vi "CRYInsert Data to Listbox.vi"(0 "OrgNames":string[](array[string]), 4 "Type":enum16{"Curves", "Values", "Results", "WFM"}(ring)=enum."Results", 6 "nData":i32[](array[numeric]), 7 "sOption":string, 8 "Waveforms":T2[](array[typedef]) {"Y dB ref" format="%.1f"; "Y axis" items=["Log", "Lin"]; "Y data" items=["dB", "Lin"]; "X data" items=["dB", "Lin"]}, 9 "Results":T3[](array[typedef]) {"Margin" format="%.2f"}, 10 "Values":T1[](array[typedef]) {"Z data" items=["dB", "Lin"]; "X data" items=["dB", "Lin"]; "Y data" items=["dB", "Lin"]; "Z dB ref" format="%.1f"; "Z axis" items=["Log", "Lin"]; "X dB ref" format="%.1f"; "X axis" items=["Log", "Lin"]; "Y axis" items=["Log", "Lin"]; "Y dB ref" format="%.1f"; "Curve"."z" format="%.2f"; "Curve"."y" format="%.2f"; "Curve"."x" format="%.2f"}, 11 "Curves":T1[](array[typedef]) {"Z data" items=["dB", "Lin"]; "X data" items=["dB", "Lin"]; "Y data" items=["dB", "Lin"]; "Z dB ref" format="%.1f"; "Z axis" items=["Log", "Lin"]; "X dB ref" format="%.1f"; "X axis" items=["Log", "Lin"]; "Y axis" items=["Log", "Lin"]; "Y dB ref" format="%.1f"; "Curve"."z" format="%.2f"; "Curve"."y" format="%.2f"; "Curve"."x" format="%.2f"}) -> (3 "Inserted Name Out":string[](array[string]))   [LabVIEW 2013]
uses:
  CRYSystem/Typedef Control/CRYData Cluster.ctl
  CRYSystem/Typedef Control/CRYResult Cluster.ctl
  CRYSystem/Typedef Control/CRYWaveform Cluster.ctl
  Global/CRYCurve Library Global.vi
  CRYProject/CRYProject Editor Global.vi
  CRYMainGlobal.vi
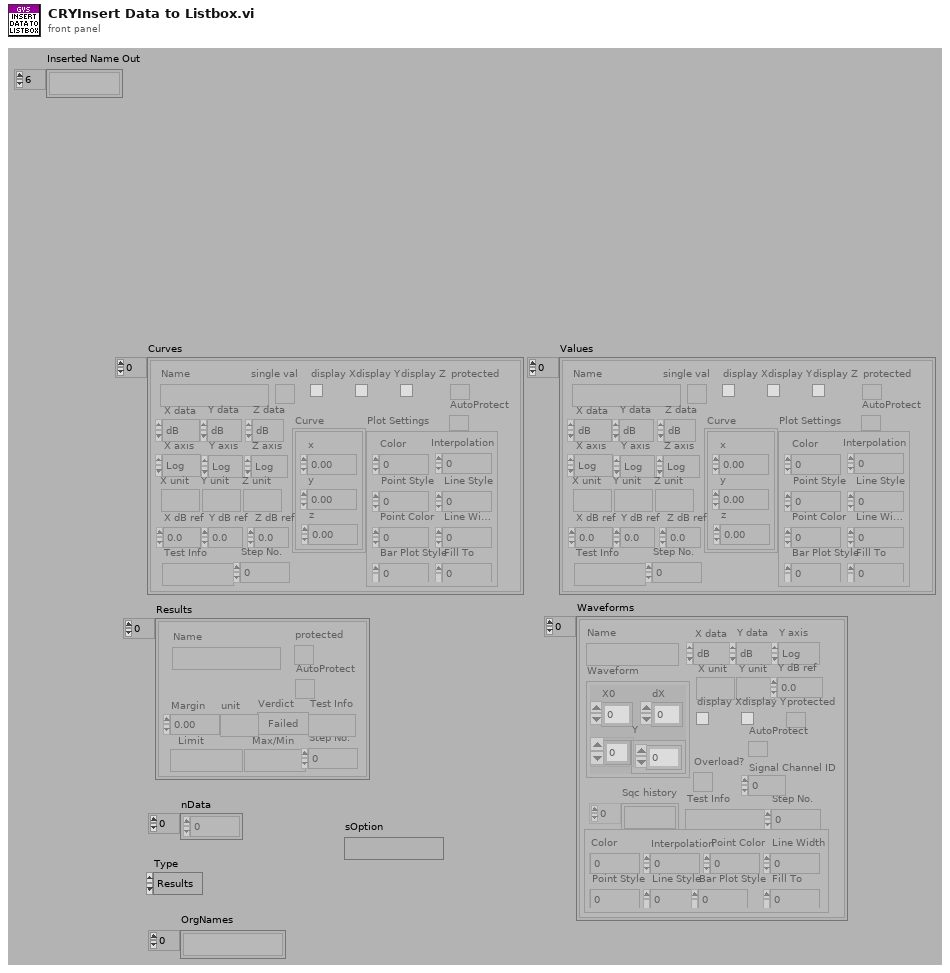
[diagram p1: front panel]
types:
  T1 = typedef "CRYData Cluster.ctl" = cluster{"Name":string, "Curve":cluster{"x":dbl, "y":dbl, "z":dbl}[], "X data":u16, "Y data":u16, "Z data":u16, "X axis":u16, "Y axis":u16, "Z axis":u16, "X unit":string, "Y unit":string, "Z unit":string, "X dB ref":dbl, "Y dB ref":dbl, "Z dB ref":dbl, "single val":bool, "protected":bool, "display X":bool, "display Y":bool, "display Z":bool, "Test Info":string, "Step No.":i32, "Plot Settings":cluster{"Color":u32, "Interpolation":u8, "Point Style":u8, "Line Style":u8, "Point Color":u32, "Line Width":u8, "Bar Plot Style":u8, "Fill To":i16}, "AutoProtect":bool}
  T2 = typedef "CRYWaveform Cluster.ctl" = cluster{"Waveform":cluster{"X0":dbl, "dX":dbl, "Y":sgl[]}, "X data":u16, "Y data":u16, "Y axis":u16, "X unit":string, "Y unit":string, "Y dB ref":dbl, "display Y":bool, "display X":bool, "Overload?":bool, "Test Info":string, "Step No.":i32, "Name":string, "protected":bool, "Sqc history":string[], "Signal Channel ID":i32, "Plot Settings":cluster{"Color":u32, "Interpolation":u8, "Point Style":u8, "Line Style":u8, "Point Color":u32, "Line Width":u8, "Bar Plot Style":u8, "Fill To":i16}, "AutoProtect":bool}
  T3 = typedef "CRYResult Cluster.ctl" = cluster{"Name":string, "Margin":dbl, "unit":string, "Verdict":bool, "Limit":string, "Max/Min":string, "protected":bool, "Step No.":i32, "Test Info":string, "AutoProtect":bool}
  T4 = typedef "CRYCurveLib Info Cluster.ctl" = cluster{"GroupingState":string}
  T5 = typedef "CRYStep.ctl" = cluster{"No.VI":i32, "Category":string, "StepName":string, "Seq setup flattened":string, "Comment":string, "Steps config.":bool[], "Jump config":i32[], "Start":dbl, "Increment":dbl, "Name":string, "Unit":string, "Y data":u16, "Y prefix":string, "Y dB ref":dbl, "Y unit":string, "Repeat State Array":cluster{"Start":dbl, "Increment":dbl, "Count":i32, "Num":i32}[]}
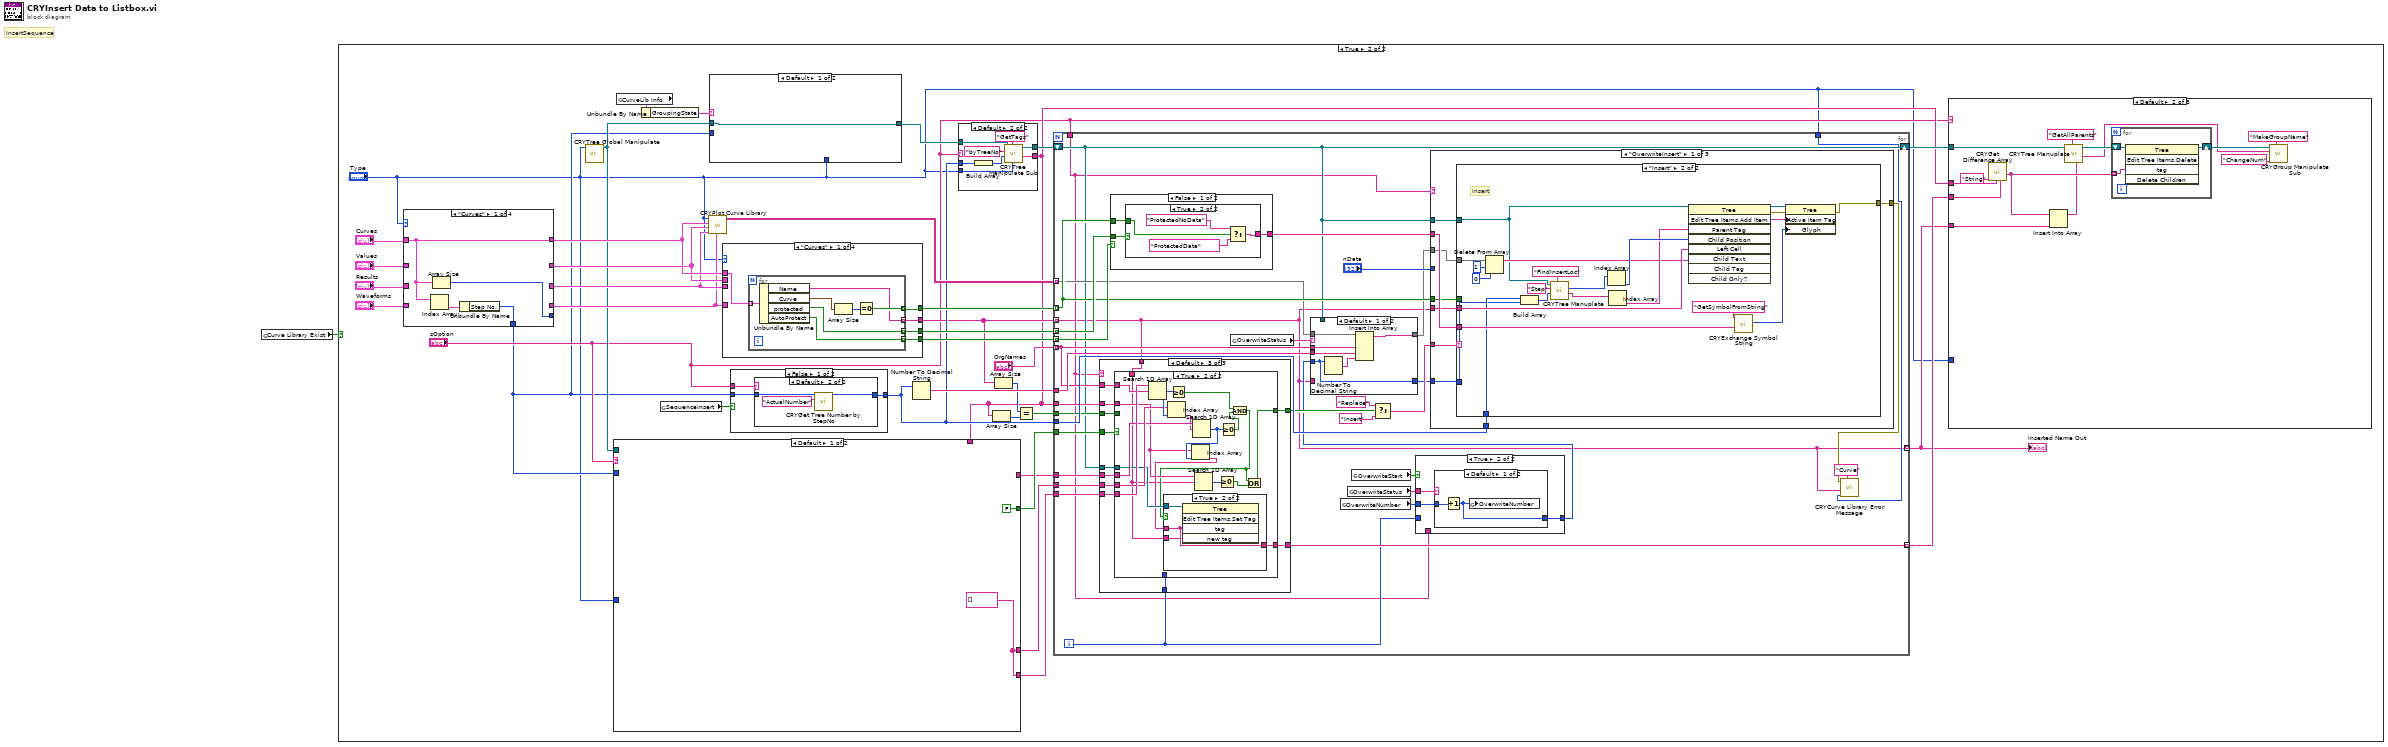
[diagram p0: block diagram]
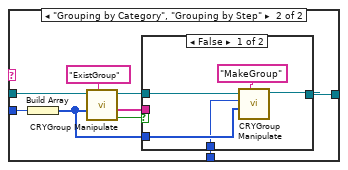
[diagram p3: hidden frame]
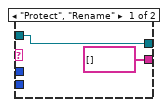
[diagram p5: hidden frame]
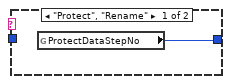
[diagram p6: hidden frame]
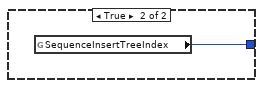
[diagram p7: hidden frame]
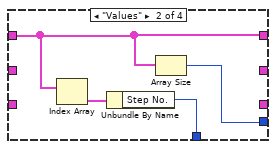
[diagram p8: hidden frame]
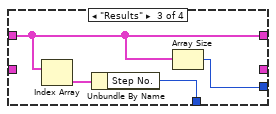
[diagram p9: hidden frame]
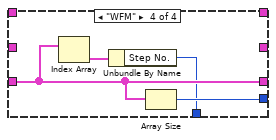
[diagram p10: hidden frame]
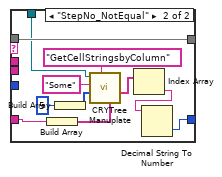
[diagram p11: hidden frame]
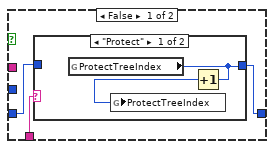
[diagram p12: hidden frame]
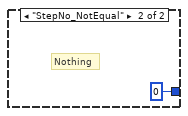
[diagram p14: hidden frame]
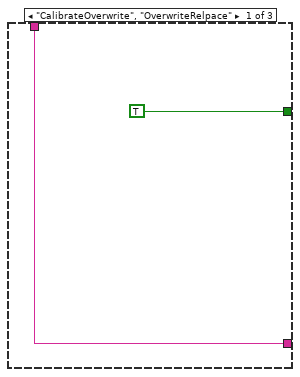
[diagram p15: hidden frame]
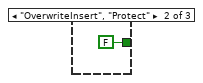
[diagram p16: hidden frame]
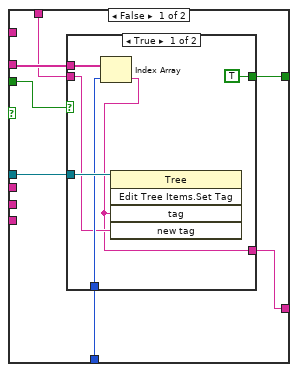
[diagram p17: hidden frame]
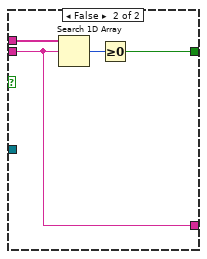
[diagram p18: hidden frame]
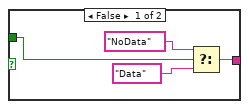
[diagram p20: hidden frame]
diagram:
  # "InsertSequence"
  n1 = global read "CRYCurve Library Global.vi" "Curve Library Exist"() -> (w1:bool)
  n2 = case shown="True" w1 {
    frame False {
    }
    frame True {
      n3 = case shown="\"Curves\"" "Type" {
        tunnel: "Curves" -> [w74 _ _ _]
        tunnel: "Results" -> [_ _ w81 _]
        tunnel: [w74 _ _ _] -> w33
        tunnel: [w75 w79 w83 w87] -> _
        tunnel: [_ _ w81 _] -> w31
        tunnel: "Waveforms" -> [_ _ _ w85]
        tunnel: [_ _ _ w85] -> w30
        tunnel: "Values" -> [_ w77 _ _]
        tunnel: [_ w77 _ _] -> w32
        tunnel: [w72 w76 w80 w84] -> w7
        frame "Curves" {
          n4 = Index Array(array=w74) -> (element=w73:T1)  [unwired: 1 in]
          n5 = Array Size(array=w74) -> (size(s)=w75:i32)
          n6 = Unbundle By Name(w73) -> ("Step No."=w72:i32)
        }
        frame "Values" {
          n7 = Index Array(array=w77) -> (element=w78:T1)  [unwired: 1 in]
          n8 = Unbundle By Name(w78) -> ("Step No."=w76:i32)
          n9 = Array Size(array=w77) -> (size(s)=w79:i32)
        }
        frame "Results" {
          n10 = Index Array(array=w81) -> (element=w82:T3)  [unwired: 1 in]
          n11 = Unbundle By Name(w82) -> ("Step No."=w80:i32)
          n12 = Array Size(array=w81) -> (size(s)=w83:i32)
        }
        frame "WFM" {
          n13 = Index Array(array=w85) -> (element=w86:T2)  [unwired: 1 in]
          n14 = Unbundle By Name(w86) -> ("Step No."=w84:i32)
          n15 = Array Size(array=w85) -> (size(s)=w87:i32)
        }
      }
      n16 = call "CRYTree Global Manipulate.vi"("Type In"="Type") -> ("Tree/Curve Tree"=w13:refnum<vi>)  [unwired: 7 in, 3 out]
      n17 = global read "CRYCurve Library Global.vi" "CurveLib Info"() -> (w9:T4)
      n18 = Unbundle By Name(w9) -> ("GroupingState"=w8:string)
      n19 = global read "CRYProject Editor Global.vi" "SequenceInsert"() -> (w14:bool)
      n20 = call "CRYPlot Curve Library.vi"("Waveform"=w30, "Results"=w31, "Values"=w32, "Curves"=w33, "Type"="Type") -> ("PlotStrings"=w34:string[][])  [unwired: 6 in]
      n21 = case shown="Default" w8 {
        tunnel: w13 -> [w38 w44]
        tunnel: [w38 w42] -> w12
        tunnel: w7 -> [_ w41]
        tunnel: "Type" -> [_ w39]
        frame Default {
        }
        frame "Grouping by Category", "Grouping by Step" {
          n22 = Build Array(w41) -> (w40:i32[])
          n23 = call "CRYGroup Manipulate.vi"("sAction"="ExistGroup", "nData"=w40, "Tree in"=w44) -> ("bData out"=w47:bool, "sData Out"=w43:string[], "Tree Out"=w46:refnum<vi>)  [unwired: 5 in, 1 out]
          n24 = case shown="False" w47 {
            tunnel: w46 -> [w51 w53]
            tunnel: w43 -> [_ _]
            tunnel: [w50 w53] -> w42
            tunnel: w40 -> [w49 _]
            tunnel: w39 -> [w48 _]
            frame False {
              n25 = call "CRYGroup Manipulate.vi"("sAction"="MakeGroup", "nData"=w49, "Type"=w48, "Tree in"=w51) -> ("Tree Out"=w50:refnum<vi>)  [unwired: 4 in, 3 out]
            }
            frame True {
            }
          }
        }
      }
      n26 = case shown="\"Curves\"" "Type" {
        tunnel: [w400 w412 w425 w439] -> w37
        tunnel: [w399 w411 w424 w438] -> w19
        tunnel: [w398 w410 w423 w437] -> w36
        tunnel: [w397 w409 w422 w436] -> w35
        tunnel: w33 -> [w396 _ _ _]
        tunnel: w32 -> [_ w408 _ _]
        tunnel: w31 -> [_ _ w421 _]
        tunnel: w30 -> [_ _ _ w435]
        frame "Curves" {
          n27 = for {
            tunnel: w396 -> [w406] mode=indexing
            tunnel: [w405] -> w400 mode=indexing
            tunnel: [w401] -> w399 mode=indexing
            tunnel: [w403] -> w398 mode=indexing
            tunnel: [w402] -> w397 mode=indexing
            n28 = Unbundle By Name(w406) -> ("Name"=w401:string, "Curve"=w407:cluster{"x":dbl, "y":dbl, "z":dbl}[], "protected"=w403:bool, "AutoProtect"=w402:bool)
            n29 = Array Size(array=w407) -> (size(s)=w404:i32)
            n30 = Equal To 0?(x=w404) -> (x = 0?=w405:bool)
          }
        }
        frame "Values" {
          n31 = for {
            tunnel: w408 -> [w419] mode=indexing
            tunnel: [w416] -> w412 mode=indexing
            tunnel: [w413] -> w411 mode=indexing
            tunnel: [w415] -> w410 mode=indexing
            tunnel: [w414] -> w409 mode=indexing
            n32 = Unbundle By Name(w419) -> ("Name"=w413:string, "Curve"=w420:cluster{"x":dbl, "y":dbl, "z":dbl}[], "protected"=w415:bool, "AutoProtect"=w414:bool)
            n33 = Array Size(array=w420) -> (size(s)=w417:i32)
            n34 = Equal?(x=w417, y=0) -> (x = y?=w416:bool)
          }
        }
        frame "Results" {
          n35 = for {
            tunnel: w421 -> [w434] mode=indexing
            tunnel: [w433] -> w425 mode=indexing
            tunnel: [w426] -> w424 mode=indexing
            tunnel: [w428] -> w423 mode=indexing
            tunnel: [w427] -> w422 mode=indexing
            n36 = Unbundle By Name(w434) -> ("Name"=w426:string, "Margin"=w432:dbl, "protected"=w428:bool, "AutoProtect"=w427:bool)
            n37 = Format Value(format string="%f", value (0)=w432) -> (output string=w429:string)  [unwired: 1 in]
            n38 = Equal?(x="NaN", y=w429) -> (x = y?=w433:bool)
          }
        }
        frame "WFM" {
          n39 = for {
            tunnel: w435 -> [w444] mode=indexing
            tunnel: [w443] -> w439 mode=indexing
            tunnel: [w440] -> w438 mode=indexing
            tunnel: [w442] -> w437 mode=indexing
            tunnel: [w441] -> w436 mode=indexing
            n40 = Unbundle By Name(w444) -> ("Name"=w440:string, "Waveform.Y"=w446:sgl[], "protected"=w442:bool, "AutoProtect"=w441:bool)
            n41 = Array Size(array=w446) -> (size(s)=w447:i32)
            n42 = Equal?(x=w447, y=0) -> (x = y?=w443:bool)
          }
        }
      }
      n43 = case shown="False" w14 {
        tunnel: "sOption" -> [w66 _]
        tunnel: [w65 w71] -> w26
        tunnel: w7 -> [w64 _]
        frame False {
          n44 = case shown="Default" w66 {
            tunnel: w64 -> [_ w70]
            tunnel: [w67 w69] -> w65
            frame "Protect", "Rename" {
              n45 = global read "CRYCurve Library Global.vi" "ProtectDataStepNo"() -> (w67:i32)
            }
            frame Default {
              n46 = call "CRYGet Tree Number by StepNo.vi"("sOption"="ActualNumber", "Step Setup VI No"=w70) -> ("Number in Tree"=w69:i32)  [unwired: 8 in, 1 out]
            }
          }
        }
        frame True {
          n47 = global read "CRYProject Editor Global.vi" "SequenceInsertTreeIndex"() -> (w71:i32)
        }
      }
      n48 = Number To Decimal String(number=w26) -> (decimal integer string=w27:string)  [unwired: 1 in]
      n49 = case shown="Default" "sOption" {
        tunnel: "Type" -> [_ w63]
        tunnel: [w55 w59] -> w29
        tunnel: w26 -> [_ w58]
        tunnel: [string[] [] ("sData Out") w57] -> w15
        tunnel: w12 -> [w55 w56]
        frame "Protect", "Rename" {
        }
        frame Default {
          n50 = Build Array(w58) -> (w60:i32[])
          n51 = call "CRYTree Manipulate Sub.vi"("Type"=w63, "sAction"="GetTags", "nData"=w60, "sOption"="byTreeNo", "Tree in"=w56) -> ("sData Out"=w57:string[], "Tree Out"=w59:refnum<vi>)  [unwired: 2 in, 3 out]
        }
      }
      n52 = case shown="Default" "sOption" {
        tunnel: w7 -> [_ w461]
        tunnel: [w448 w460] -> w23
        tunnel: [FALSE w459] -> w25
        tunnel: [w448 w458] -> w22
        tunnel: w13 -> [_ w455]
        tunnel: [_ w452] -> w21
        tunnel: "Type" -> [_ w451]
        tunnel: w15 -> [_ w450]
        frame Default {
          w448 = string[] [] ("Changed Curve State")
        }
        frame "Apply", "StepOK" {
          n53 = call "CRYGet Current TS Steps.vi"() -> ("Steps"=w462:T5[])  [unwired: 7 in, 4 out]
          n54 = for {
            tunnel: w462 -> [w509] mode=indexing
            tunnel: w461 -> [w507]
            tunnel: [w502] -> w459
            stop <- w502 stop-if-true
            n55 = Unbundle By Name(w509) -> ("No.VI"=w508:i32, "Category"=w505:string)
            n56 = Equal?(x=w507, y=w508) -> (x = y?=w506:bool)
            n57 = Equal?(x=w505, y="Analysis") -> (x = y?=w500:bool)
            n58 = Equal?(x=w505, y="Acqusition") -> (x = y?=w501:bool)
            n59 = Or(x=w500, y=w501) -> (x .or. y?=w499:bool)
            n60 = And(x=w506, y=w499) -> (x .and. y?=w502:bool)
          }
          n61 = case shown="True" w459 {
            tunnel: [_ w463] -> w460
            tunnel: [_ w464] -> w458
            tunnel: w451 -> [_ w467]
            frame False {
            }
            frame True {
              w465 = string[] [] ("Changed Curve State")
              n62 = global read "CRYMainGlobal.vi" "Changed Curve State"() -> (w466:string[][])
              n63 = for {
                tunnel: w467 -> [w486]
                tunnel: w466 -> [w481] mode=indexing
                shift-right: [w470] -> w464
                shift-left: w465 -> [w471]
                shift-right: [w468] -> w463
                shift-left: w465 -> [w469]
                # "New Names"
                # "Old Names"
                n64 = case shown="\"WFM\"" w486 {
                  tunnel: ["Curve" ("Custom Curve Names") "Value" ("Custom Curve Names") "Result" ("Custom Curve Names") "Wave" ("Custom Curve Names")] -> w480
                  frame "Curves", Default {
                  }
                  frame "Values" {
                  }
                  frame "Results" {
                  }
                  frame "WFM" {
                  }
                }
                n65 = Index Array(array=w481, index #1=3 ("index"), index #2=2 ("index"), index #3=0 ("index"), index #4=1 ("index")) -> (element #1=w479:string, element #2=w478:string, element #3=w473:string, element #4=w472:string)
                n66 = Equal?(x=w480, y=w479) -> (x = y?=w476:bool)
                n67 = Equal?(x="R", y=w478) -> (x = y?=w475:bool)
                n68 = And(x=w476, y=w475) -> (x .and. y?=w474:bool)
                n69 = case shown="True" w474 {
                  tunnel: w473 -> [_ w490]
                  tunnel: w472 -> [_ w489]
                  tunnel: w471 -> [w488 w494]
                  tunnel: [w488 w493] -> w470
                  tunnel: w469 -> [w487 w492]
                  tunnel: [w487 w491] -> w468
                  frame False {
                  }
                  frame True {
                    n70 = Insert Into Array(array=w492, new element=w489) -> (w491:string[])  [unwired: 1 in]
                    n71 = Insert Into Array(array=w494, new element=w490) -> (w493:string[])  [unwired: 1 in]
                  }
                }
              }
            }
          }
          n72 = Build Array(3) -> (w453:i32[])
          n73 = call "CRYTree Manuplate.vi"("sData"=w450, "sAction"="GetCellStringsbyColumn", "nData"=w453, "sOption"="Some", "Tree in"=w455) -> ("sData Out"=w452:string[])  [unwired: 3 in, 3 out]
        }
      }
      n74 = Array Size(array=w15) -> (size(s)=w17:i32)
      n75 = Array Size(array=w19) -> (size(s)=w18:i32)
      n76 = Equal?(x=w18, y=w17) -> (x = y?=w16:bool)
      n77 = for {
        tunnel: [w89] -> w10 mode=indexing
        tunnel: w34 -> [w95] mode=indexing
        tunnel: w37 -> [w119] mode=indexing
        tunnel: w19 -> [w89] mode=indexing
        tunnel: w36 -> [w120] mode=indexing
        tunnel: w35 -> [w121] mode=indexing
        shift-right: [w93] -> w28
        shift-left: w29 -> [w93]
        tunnel: "OrgNames" -> [w109] mode=indexing
        tunnel: w27 -> [w117]
        tunnel: w26 -> [w113]
        tunnel: w15 -> [w105]
        tunnel: "sOption" -> [w92]
        tunnel: w25 -> [w110]
        tunnel: w23 -> [w107]
        tunnel: w22 -> [w108]
        tunnel: w21 -> [w106]
        tunnel: [w104] -> w20 mode=indexing
        tunnel: w16 -> [w103]
        tunnel: "Type" -> [w90]
        i -> [w99]
        n78 = case shown="Default" w92 {
          tunnel: w105 -> [_ _ w159]
          tunnel: w89 -> [w151 _ w158]
          tunnel: [TRUE FALSE w157] -> w112
          tunnel: w110 -> [_ _ w165]
          tunnel: w109 -> [_ _ w164]
          tunnel: w108 -> [_ _ w163]
          tunnel: w107 -> [_ _ w162]
          tunnel: w106 -> [_ _ w161]
          tunnel: w93 -> [_ _ w160]
          tunnel: [w151 _ w156] -> w104
          tunnel: w103 -> [_ _ w155]
          tunnel: w99 -> [_ _ w154]
          frame "CalibrateOverwrite", "OverwriteRelpace" {
          }
          frame "OverwriteInsert", "Protect" {
          }
          frame Default {
            n79 = case shown="True" w165 {
              tunnel: w159 -> [w172 w188]
              tunnel: w158 -> [w170 w184]
              tunnel: w164 -> [_ w199]
              tunnel: w163 -> [_ w197]
              tunnel: w162 -> [_ w200]
              tunnel: w161 -> [_ w195]
              tunnel: w160 -> [w169 w191]
              tunnel: [w171 w185] -> w157
              tunnel: [w166 w183] -> w156
              tunnel: w155 -> [w168 _]
              tunnel: w154 -> [w167 _]
              frame False {
                n80 = case shown="True" w168 {
                  tunnel: w172 -> [w176 w181]
                  tunnel: [TRUE w180] -> w171
                  tunnel: w170 -> [w174 w179]
                  tunnel: w169 -> [w178 _]
                  tunnel: w167 -> [w175 _]
                  tunnel: [w173 w179] -> w166
                  frame True {
                    n81 = Index Array(array=w176, index=w175) -> (element=w173:string)
                    n82 = invoke class="Tree" method="Edit Tree Items.Set Tag"(reference=w178, "tag"=w173, "new tag"=w174) -> ()  [unwired: 2 in, 5 out]
                  }
                  frame False {
                    n83 = Search 1D Array(1D array=w181, element=w179) -> (index of element=w182:i32)  [unwired: 1 in]
                    n84 = Greater Or Equal To 0?(x=w182) -> (x >= 0?=w180:bool)
                  }
                }
              }
              frame True {
                n85 = Search 1D Array(1D array=w200, element=w199) -> (index of element=w198:i32)  [unwired: 1 in]
                n86 = Index Array(array=w197, index=w198) -> (element=w194:string)
                n87 = Greater Or Equal To 0?(x=w198) -> (x >= 0?=w196:bool)
                n88 = Search 1D Array(1D array=w195, element=w194) -> (index of element=w192:i32)  [unwired: 1 in]
                n89 = Index Array(array=w188, index=w192) -> (element=w190:string)
                n90 = Search 1D Array(1D array=w188, element=w184) -> (index of element=w189:i32)  [unwired: 1 in]
                n91 = Greater Or Equal To 0?(x=w189) -> (x >= 0?=w187:bool)
                n92 = Greater Or Equal To 0?(x=w192) -> (x >= 0?=w193:bool)
                n93 = And(x=w196, y=w193) -> (x .and. y?=w186:bool)
                n94 = case shown="True" w186 {
                  tunnel: w191 -> [_ w204]
                  tunnel: w190 -> [_ w203]
                  tunnel: w184 -> [w201 w202]
                  tunnel: [w201 w203] -> w183
                  frame False {
                  }
                  frame True {
                    n95 = invoke class="Tree" method="Edit Tree Items.Set Tag"(reference=w204, "tag"=w203, "new tag"=w202) -> ()  [unwired: 2 in, 5 out]
                  }
                }
                n96 = Or(x=w186, y=w187) -> (x .or. y?=w185:bool)
              }
            }
          }
        }
        n97 = case shown="False" w121 {
          tunnel: w119 -> [w206 w219]
          tunnel: [w205 w218] -> w118
          tunnel: w120 -> [w207 _]
          frame False {
            n98 = case shown="True" w207 {
              tunnel: w206 -> [w211 w215]
              tunnel: [w210 w214] -> w205
              frame False {
                n99 = Select(t="NoData" ("name or relative path"), s=w211, f="Data" ("name or relative path")) -> (s? t:f=w210:string)
              }
              frame True {
                n100 = Select(t="ProtectedNoData" ("name or relative path"), s=w215, f="ProtectedData" ("name or relative path")) -> (s? t:f=w214:string)
              }
            }
          }
          frame True {
            # "AutoProtect"
            n101 = Select(t="AutoProtectNoData" ("name or relative path"), s=w219, f="AutoProtectData" ("name or relative path")) -> (s? t:f=w218:string)
          }
        }
        n102 = global read "CRYCurve Library Global.vi" "OverwriteStatus"() -> (w97:string)
        n103 = global read "CRYCurve Library Global.vi" "OverwriteNumber"() -> (w100:i32)
        n104 = global read "CRYCurve Library Global.vi" "OverwriteStatus"() -> (w101:string)
        n105 = global read "CRYCurve Library Global.vi" "OverwriteStart"() -> (w102:bool)
        n106 = Select(t="Replace", s=w112, f="Insert" ("sOption")) -> (s? t:f=w114:string)
        n107 = case shown="True" w102 {
          tunnel: w101 -> [_ w147]
          tunnel: w100 -> [_ w146]
          tunnel: w99 -> [w140 _]
          tunnel: [w141 w145] -> w98
          tunnel: w92 -> [w139 _]
          frame False {
            n108 = case shown="\"Protect\"" w139 {
              tunnel: [w143 w144] -> w141
              tunnel: w140 -> [_ w144]
              frame "Protect" {
                n109 = global read "CRYCurve Library Global.vi" "ProtectTreeIndex"() -> (w143:i32)
                n110 = Increment(x=w143) -> (x+1=w142:i32)
                n111 = global write "CRYCurve Library Global.vi" "ProtectTreeIndex"(w142) -> ()
              }
              frame Default {
              }
            }
          }
          frame True {
            n112 = case shown="Default" w147 {
              tunnel: w146 -> [w149 _]
              tunnel: [w148 0] -> w145
              frame Default {
                n113 = Increment(x=w149) -> (x+1=w148:i32)
                n114 = global write "CRYCurve Library Global.vi" "OverwriteNumber"(w148) -> ()
              }
              frame "StepNo_NotEqual" {
                # "Nothing"
              }
            }
          }
        }
        n115 = case shown="Default" w97 {
          tunnel: w117 -> [w127 _]
          tunnel: w109 -> [w125 _]
          tunnel: w98 -> [w122 _]
          tunnel: [w124 w138] -> w96
          tunnel: w95 -> [w123 w138]
          tunnel: [w122 w128] -> w94
          tunnel: w89 -> [_ w133]
          tunnel: w93 -> [_ w131]
          frame Default {
            n116 = Number To Decimal String(number=w122) -> (decimal integer string=w126:string)  [unwired: 1 in]
            n117 = Insert Into Array(array=w123, new element #1=w125, new element #2=w127, new element #3=w126) -> (w124:string[])  [unwired: 1 in]
          }
          frame "StepNo_NotEqual" {
            n118 = Build Array(w133) -> (w132:string[])
            n119 = Build Array(5) -> (w134:i32[])
            n120 = call "CRYTree Manuplate.vi"("sData"=w132, "sAction"="GetCellStringsbyColumn", "nData"=w134, "sOption"="Some", "Tree in"=w131) -> ("sData Out"=w130:string[])  [unwired: 3 in, 3 out]
            n121 = Index Array(array=w130) -> (element=w129:string)  [unwired: 1 in]
            n122 = Decimal String To Number(string=w129) -> (number=w128:i32)  [unwired: 2 in, 1 out]
          }
        }
        n123 = case shown="\"OverwriteInsert\"" w92 {
          tunnel: w118 -> [w228 w295 _]
          tunnel: w96 -> [w227 w294 w381]
          tunnel: w119 -> [w226 w293 _]
          tunnel: w114 -> [w222 w292 _]
          tunnel: w93 -> [w225 w291 w383]
          tunnel: w89 -> [w224 w290 _]
          tunnel: w113 -> [w223 w289 _]
          tunnel: "nData" -> [_ _ w386]
          tunnel: w94 -> [w221 w288 w380]
          tunnel: [w220 w287 w377] -> w91
          frame "OverwriteInsert" {
            n124 = case shown="\"Insert\"" w222 {
              tunnel: w227 -> [w237 w269]
              tunnel: w228 -> [w242 w282]
              tunnel: w226 -> [w244 _]
              tunnel: w225 -> [w243 w267]
              tunnel: w224 -> [w232 w284]
              tunnel: w223 -> [_ w280]
              tunnel: w221 -> [_ w279]
              tunnel: [w229 w265] -> w220
              frame "Replace", Default {
                n125 = property on="Property Node" class="Tree"(reference=w243, "Active Item Tag"=w232) -> (reference out=w240:refnum<vi>, error out=w231:errorcluster, "Glyph"=w239:i32)  [unwired: 1 in]
                n126 = call "CRYExchange Symbol String.vi"("nData"=w239, "sAction"="GetStringFromSymbol") -> ("sData out"=w235:string)  [unwired: 8 in, 1 out]
                n127 = case shown="\"DataView\", \"NoDataView\"" w235 {
                  tunnel: w244 -> [_ w249 w253 w257]
                  tunnel: [w245 w248 w252 w256] -> w233
                  tunnel: w242 -> [w245 _ _ _]
                  frame Default {
                  }
                  frame "DataView", "NoDataView" {
                    n128 = Select(t="NoDataView" ("name or relative path"), s=w249, f="DataView" ("name or relative path")) -> (s? t:f=w248:string)
                  }
                  frame "AutoProtectDataView", "AutoProtectNoDataView" {
                    n129 = Select(t="AutoProtectNoDataView" ("name or relative path"), s=w253, f="AutoProtectDataView" ("name or relative path")) -> (s? t:f=w252:string)
                  }
                  frame "ProtectedDataView", "ProtectedNoDataView" {
                    n130 = Select(t="ProtectedNoDataView" ("name or relative path"), s=w257, f="ProtectedDataView" ("name or relative path")) -> (s? t:f=w256:string)
                  }
                }
                n131 = call "CRYExchange Symbol String.vi"("sData"=w233, "sAction"="GetSymbolFromString") -> ("nData out"=w238:i32)  [unwired: 8 in, 1 out]
                n132 = property on="Property Node" class="Tree"(reference=w240, error in=w231, "Active Item Tag"=w232, "Glyph"=w238) -> (reference out=w241:refnum<vi>, error out=w230:errorcluster)
                n133 = for {
                  shift-right: [w263] -> _
                  shift-left: w241 -> [w264]
                  tunnel: w232 -> [w262]
                  tunnel: w237 -> [w260] mode=indexing
                  shift-right: [w258] -> w229
                  shift-left: w230 -> [w259]
                  i -> [w261]
                  n134 = property on="Property Node" class="Tree"(reference=w264, error in=w259, "Active Item Tag"=w262, "ActiveColNum"=w261, "Cell String"=w260) -> (reference out=w263:refnum<vi>, error out=w258:errorcluster)
                }
              }
              frame "Insert" {
                # "Insert"
                n135 = Delete From Array(array=w269, length=1, index=0) -> (array with subset deleted=w268:string[])  [unwired: 1 out]
                n136 = Build Array(w280, w279) -> (w274:i32[])
                n137 = call "CRYTree Manuplate.vi"("sAction"="FindInsertLoc", "nData"=w274, "sOption"="Step", "Tree in"=w267) -> ("sData Out"=w275:string[], "nData Out"=w276:i32[])  [unwired: 4 in, 2 out]
                n138 = Index Array(array=w276) -> (element=w273:i32)  [unwired: 1 in]
                n139 = Index Array(array=w275) -> (element=w272:string)  [unwired: 1 in]
                n140 = invoke class="Tree" method="Edit Tree Items.Add Item"(reference=w267, "Parent Tag"=w272, "Child Position"=w273, "Left Cell"=w284, "Child Text"=w268) -> (reference out=w285:refnum<vi>, error out=w266:errorcluster, "Edit Tree Items:Add Item"=w286:string)  [unwired: 4 in, 6 out]
                n141 = call "CRYExchange Symbol String.vi"("sData"=w282, "sAction"="GetSymbolFromString") -> ("nData out"=w281:i32)  [unwired: 8 in, 1 out]
                n142 = property class="Tree"(reference=w285, error in=w266, "Active Item Tag"=w286, "Glyph"=w281) -> (error out=w265:errorcluster)  [unwired: 1 out]
              }
            }
          }
          frame Default {
            n143 = case shown="\"Replace\"" w292 {
              tunnel: w294 -> [w318 w363]
              tunnel: w295 -> [w322 w372]
              tunnel: w293 -> [w323 _]
              tunnel: w291 -> [w308 w370]
              tunnel: w290 -> [w297 w374]
              tunnel: w289 -> [w312 w366]
              tunnel: w288 -> [w305 w361]
              tunnel: [w296 w354] -> w287
              frame "Replace" {
                n144 = Build Array(w312, w305) -> (w317:i32[])
                n145 = Build Array(w297) -> (w309:string[])
                n146 = call "CRYTree Manuplate.vi"("sData"=w309, "sAction"="FindInsertLoc", "nData"=w317, "sOption"="MovebyReplace", "Tree in"=w308) -> ("bResult Out"=w311:bool, "sData Out"=w316:string[], "nData Out"=w315:i32[], "Tree Out"=w306:refnum<vi>)  [unwired: 3 in]
                n147 = property on="Property Node" class="Tree"(reference=w306, "Active Item Tag"=w297) -> (reference out=w310:refnum<vi>, error out=w300:errorcluster, "Glyph"=w320:i32)  [unwired: 1 in]
                n148 = call "CRYExchange Symbol String.vi"("nData"=w320, "sAction"="GetStringFromSymbol") -> ("sData out"=w303:string)  [unwired: 8 in, 1 out]
                n149 = case shown="\"ProtectedDataView\", \"ProtectedNoDataView\"" w303 {
                  tunnel: w323 -> [_ w328 w332 w336]
                  tunnel: [w324 w327 w331 w335] -> w301
                  tunnel: w322 -> [w324 _ _ _]
                  frame Default {
                  }
                  frame "DataView", "NoDataView" {
                    n150 = Select(t="NoDataView" ("name or relative path"), s=w328, f="DataView" ("name or relative path")) -> (s? t:f=w327:string)
                  }
                  frame "AutoProtectDataView", "AutoProtectNoDataView" {
                    n151 = Select(t="AutoProtectNoDataView" ("name or relative path"), s=w332, f="AutoProtectDataView" ("name or relative path")) -> (s? t:f=w331:string)
                  }
                  frame "ProtectedDataView", "ProtectedNoDataView" {
                    n152 = Select(t="ProtectedNoDataView" ("name or relative path"), s=w336, f="ProtectedDataView" ("name or relative path")) -> (s? t:f=w335:string)
                  }
                }
                n153 = call "CRYExchange Symbol String.vi"("sData"=w301, "sAction"="GetSymbolFromString") -> ("nData out"=w319:i32)  [unwired: 8 in, 1 out]
                n154 = property on="Property Node" class="Tree"(reference=w310, error in=w300, "Active Item Tag"=w297, "Glyph"=w319) -> (reference out=w321:refnum<vi>, error out=w299:errorcluster)
                n155 = for {
                  shift-right: [w352] -> w307
                  shift-left: w321 -> [w353]
                  tunnel: w297 -> [w351]
                  tunnel: w318 -> [w349] mode=indexing
                  shift-right: [w347] -> w298
                  shift-left: w299 -> [w348]
                  i -> [w350]
                  n156 = property on="Property Node" class="Tree"(reference=w353, error in=w348, "Active Item Tag"=w351, "ActiveColNum"=w350, "Cell String"=w349) -> (reference out=w352:refnum<vi>, error out=w347:errorcluster)
                }
                n157 = case shown="False" w311 {
                  tunnel: w316 -> [w345 _]
                  tunnel: w315 -> [w344 _]
                  tunnel: w297 -> [w341 _]
                  tunnel: w307 -> [w339 _]
                  tunnel: w298 -> [w338 w346]
                  tunnel: [w337 w346] -> w296
                  frame False {
                    n158 = Index Array(array=w345) -> (element=w342:string)  [unwired: 1 in]
                    n159 = Index Array(array=w344) -> (element=w343:i32)  [unwired: 1 in]
                    n160 = invoke class="Tree" method="Edit Tree Items.Move Item"(reference=w339, error in=w338, "tag"=w341, "New Parent"=w342, "New Position"=w343, "Carry Children"=TRUE ("Carry Children?")) -> (error out=w337:errorcluster)  [unwired: 1 in, 6 out]
                  }
                  frame True {
                  }
                }
              }
              frame "Insert", Default {
                n161 = Build Array(w366, w361) -> (w356:i32[])
                n162 = call "CRYTree Manuplate.vi"("sAction"="FindInsertLoc", "nData"=w356, "sOption"="Step", "Tree in"=w370) -> ("sData Out"=w357:string[], "nData Out"=w358:i32[], "Tree Out"=w369:refnum<vi>)  [unwired: 4 in, 1 out]
                n163 = Delete From Array(array=w363, length=1, index=0) -> (array with subset deleted=w362:string[])  [unwired: 1 out]
                n164 = Index Array(array=w358) -> (element=w367:i32)  [unwired: 1 in]
                n165 = Index Array(array=w357) -> (element=w368:string)  [unwired: 1 in]
                n166 = invoke class="Tree" method="Edit Tree Items.Add Item"(reference=w369, "Parent Tag"=w368, "Child Position"=w367, "Left Cell"=w374, "Child Text"=w362) -> (reference out=w375:refnum<vi>, error out=w355:errorcluster, "Edit Tree Items:Add Item"=w376:string)  [unwired: 4 in, 6 out]
                n167 = call "CRYExchange Symbol String.vi"("sData"=w372, "sAction"="GetSymbolFromString") -> ("nData out"=w371:i32)  [unwired: 8 in, 1 out]
                n168 = property class="Tree"(reference=w375, error in=w355, "Active Item Tag"=w376, "Glyph"=w371) -> (error out=w354:errorcluster)  [unwired: 1 out]
              }
            }
          }
          frame "Rename" {
            # "Rename in CRYRename All.vi"
            n169 = Index Array(array=w386, index=w380) -> (element=w385:i32)
            n170 = property on="Property Node" class="Tree"(reference=w383, "Active Item Row Number"=w385) -> (reference out=w382:refnum<vi>, error out=w379:errorcluster, "Active Item Tag"=w384:string)  [unwired: 1 in]
            n171 = Index Array(array=w381) -> (element=w387:string)  [unwired: 1 in]
            n172 = for {
              shift-right: [w394] -> w388
              shift-left: w382 -> [w395]
              tunnel: w384 -> [w393]
              tunnel: w381 -> [w391] mode=indexing
              shift-right: [w389] -> w378
              shift-left: w379 -> [w390]
              i -> [w392]
              n173 = property on="Property Node" class="Tree"(reference=w395, error in=w390, "Active Item Tag"=w393, "ActiveColNum"=w392, "Cell String"=w391) -> (reference out=w394:refnum<vi>, error out=w389:errorcluster)
            }
            n174 = invoke class="Tree" method="Edit Tree Items.Set Tag"(reference=w388, error in=w378, "tag"=w384, "new tag"=w387) -> (error out=w377:errorcluster)  [unwired: 1 in, 4 out]
          }
        }
        n175 = call "CRYCurve Library Error Message.vi"("sAction"="Curve", "Type"=w90, "sData"=w89, "error IO"=w91) -> ()  [unwired: 8 in]
      }
      "Inserted Name Out" <- w10
      n176 = case shown="Default" "sOption" {
        tunnel: w28 -> [_ w518 w528]
        tunnel: w20 -> [_ w522 _]
        tunnel: w15 -> [_ w521 _]
        tunnel: w10 -> [_ w511 w529]
        tunnel: "Type" -> [_ _ _]
        frame "CalibrateOverwrite", "OverwriteInsert", "OverwriteRelpace", "Rename" {
          # "None"
        }
        frame Default {
          n177 = call "CRYGet Difference Array.vi"("String2"=w522, "String1"=w521, "sOption"="String") -> ("StringDiff Out"=w512:string[])  [unwired: 7 in, 1 out]
          n178 = Insert Into Array(array=w512, new element=w511) -> (w510:string[])  [unwired: 1 in]
          n179 = call "CRYTree Manuplate.vi"("sData"=w510, "sAction"="GetAllParents", "Tree in"=w518) -> ("sData Out"=w513:string[], "Tree Out"=w517:refnum<vi>)  [unwired: 5 in, 2 out]
          n180 = for {
            tunnel: w512 -> [w524] mode=indexing
            shift-right: [w523] -> w514
            shift-left: w517 -> [w525]
            n181 = invoke class="Tree" method="Edit Tree Items.Delete"(reference=w525, "tag"=w524) -> (reference out=w523:refnum<vi>)  [unwired: 3 in, 4 out]
          }
          n182 = call "CRYGroup Manipulate Sub.vi"("sAction"="MakeGroupName", "sOption"="ChangeNum", "sData"=w513, "Tree in"=w514) -> ()  [unwired: 3 in, 5 out]
        }
        frame "Protect" {
          n183 = Index Array(array=w529) -> (element=w527:string)  [unwired: 1 in]
          n184 = Empty String/Path?(string/path=w527) -> (empty?=w526:bool)
          n185 = case shown="False" w526 {
            tunnel: w527 -> [w534 _]
            tunnel: w528 -> [w531 _]
            frame False {
              n186 = invoke class="Tree" method="Navigate Tree.Get Parent"(reference=w531, "tag"=w534) -> (reference out=w533:refnum<vi>, "Navigate Tree:Get Parent"=w532:string)  [unwired: 2 in, 2 out]
              n187 = Build Array(w532) -> (w530:string[])
              n188 = call "CRYGroup Manipulate Sub.vi"("sAction"="MakeGroupName", "sOption"="ChangeNum", "sData"=w530, "Tree in"=w533) -> ()  [unwired: 3 in, 5 out]
            }
            frame True {
            }
          }
        }
      }
    }
  }
